vi "Get Owning Task.vi"(8 "error in (no error)":errorcluster, 11 "Group Config in":refnum<class "Group Config.lvclass">) -> (0 "error out":errorcluster, 2 "Task":string, 3 "Group Config out":refnum<class "Group Config.lvclass">)   [LabVIEW 2020, in "Vecto.lvlib" / "Group Config.lvclass"]
uses:
  Group Config.lvclass
  Group Config.lvclass/Group Config.ctl
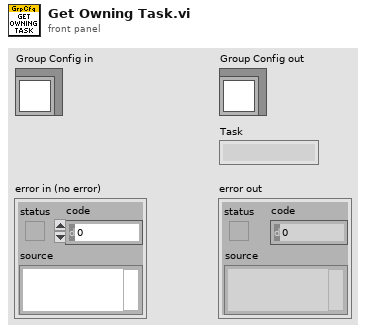
[diagram p1: front panel]
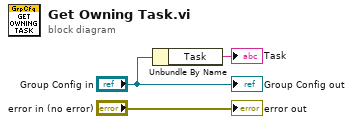
[diagram p0: block diagram]
diagram:
  n1 = Unbundle By Name("Group Config in") -> ("Task"=→"Task":string)
  "error out" <- "error in (no error)"
  "Group Config out" <- "Group Config in"
